vi "Mining Routine.vi"(9 "Blocks to find":i32=1, 10 "camera params":T4, 11 "FPGA VI Reference In":T1) -> (2 "Timed out":bool)   [LabVIEW 2012]
uses:
  <vilib>/vision/Image Controls.llb/IMAQ Image.ctl
  <vilib>/httpClient/ClientHandle.ctl
  FPGA_ref.ctl
  Globals.vi
  <vilib>/httpClient/LabVIEWHTTPClient.lvlib
panel:
  in  "Timeout (ms)":u32=120000
  in  "Block forward \ntime (10ms)":i32=300
  in  "Forward safe distance":dbl=0.35
  in  "No block distance":dbl=0.5
  in  "Block pickup distance":dbl=0.35
  in  "Block Y-Offset":dbl=400.0
  in  "Block X-Offset":dbl=160.0
  in  "Camera turn speed":dbl=0.25
  in  "Block Mid Range":dbl=50.0
  in  "no block turn speed":dbl=0.3
  # "Complete mining routine to search for & collect blocks\n\nWill exit when all blocks are found, or timeout occours"
  # "Not calibrated. Guessed.."
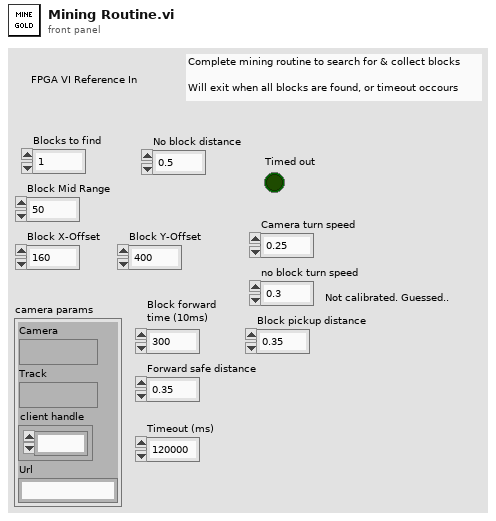
[diagram p1: front panel]
types:
  T1 = typedef "FPGA_ref.ctl" = refnum<k20>
  T2 = typedef "IMAQ Image.ctl" = refnum<image>
  T3 = typedef "LabVIEWHTTPClient.lvlib/ClientHandle.ctl" = refnum<k1>
  T4 = cluster{"Camera":T2, "Track":T2, "client handle":T3, "Url":string}
  T5 = cluster{"X Velocity (m/s)":dbl, "Y Velocity (m/s)":dbl, "Angular Velocity (rad/s)":dbl}
  T6 = cluster{"Blocks picked up":i32, "Timeout":i32, "Next state":enum16{"start", "find block", "align block", "pickup block", "sort block", "finish"}, "Future state":enum16{"start", "find block", "align block", "pickup block", "sort block", "finish"}, "Blocks to find":i32}
  T7 = enum16{"start", "find block", "align block", "pickup block", "sort block", "finish"}
  T8 = enum16{"position", "arm down", "forward", "grab", "arm up"}
  T9 = enum16{"wait", "open", "close", "lift", "lower", "pickup", "Flip", "UnFlip", "Latch", "UnLatch", "Setup"}
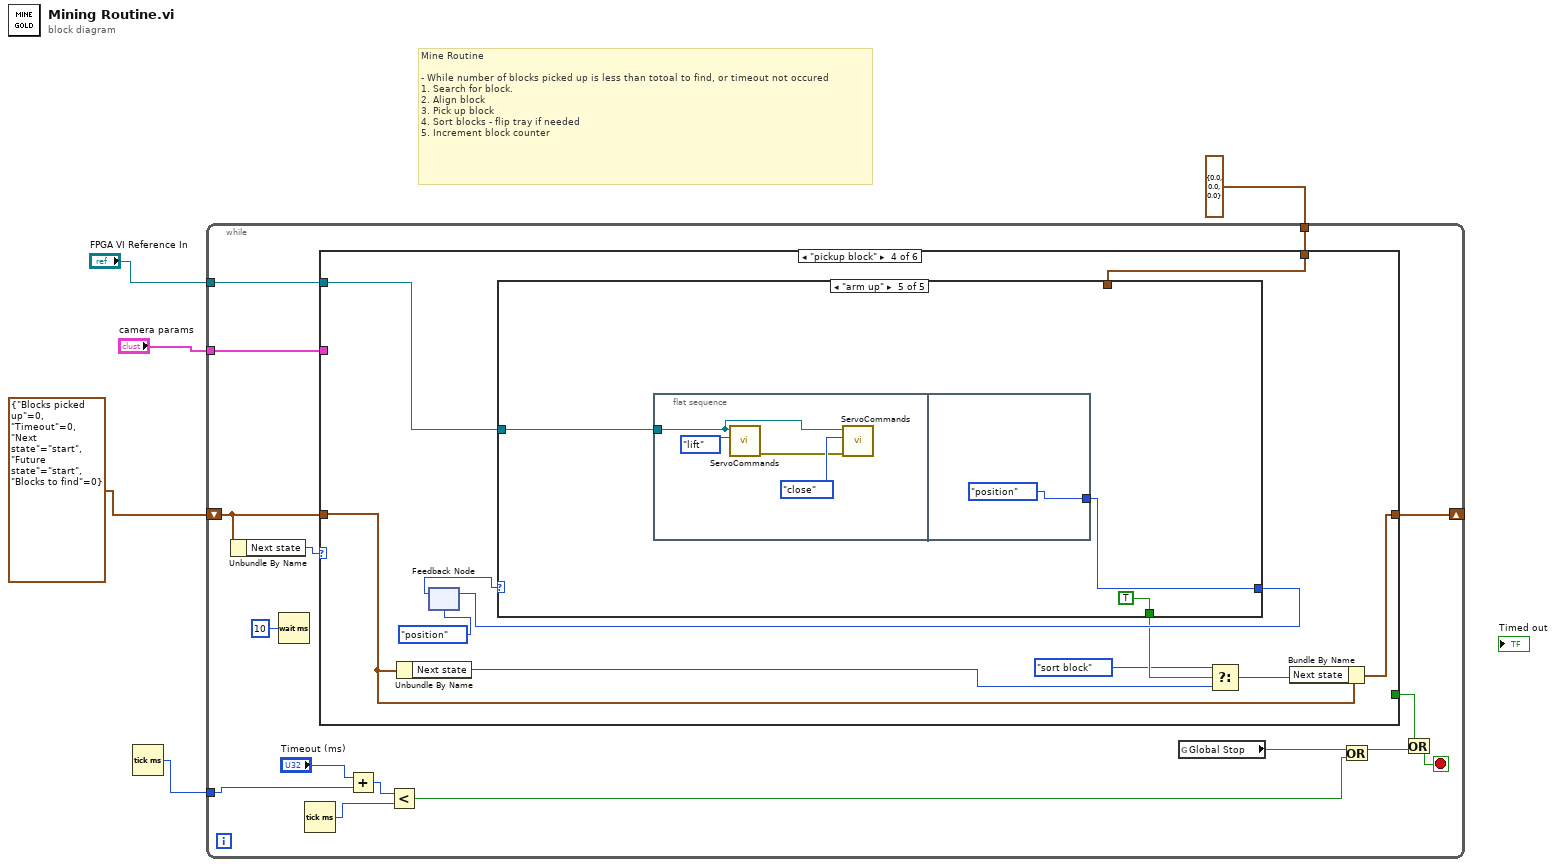
[diagram p0: block diagram]
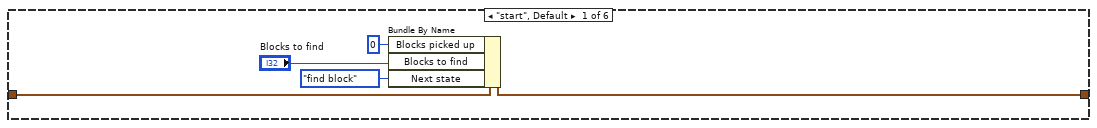
[diagram p2: hidden frame]
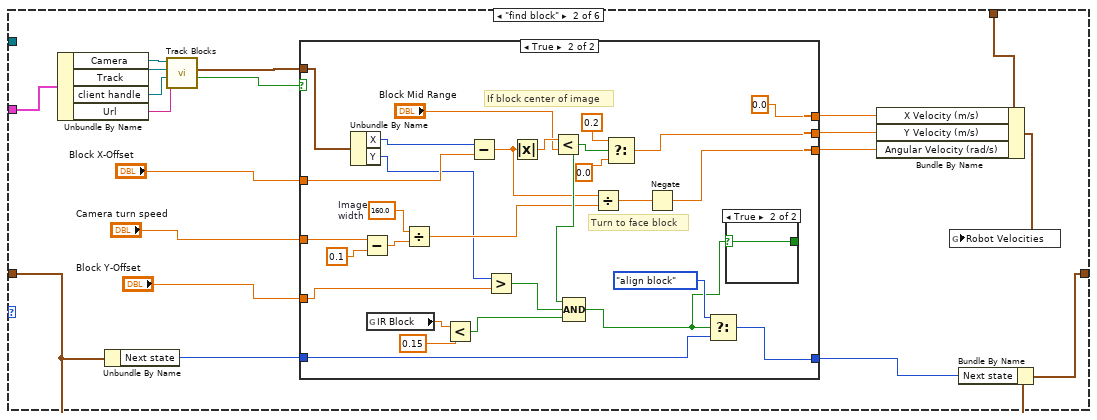
[diagram p3: hidden frame]
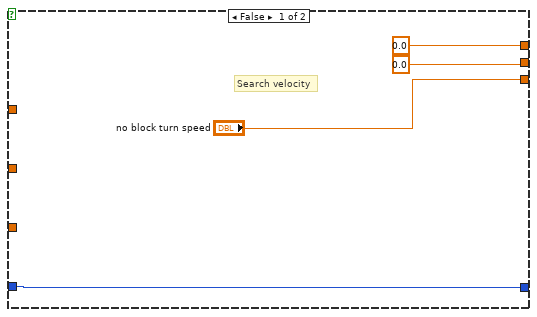
[diagram p4: hidden frame]
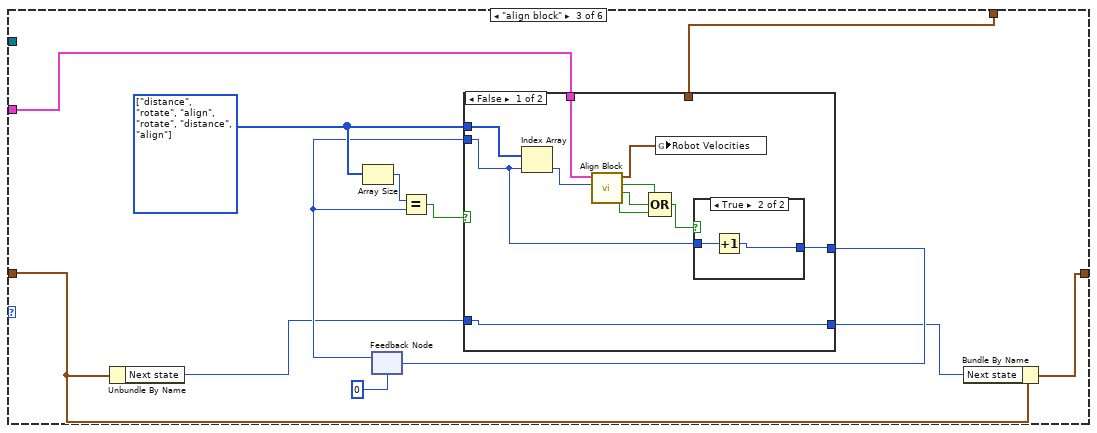
[diagram p6: hidden frame]
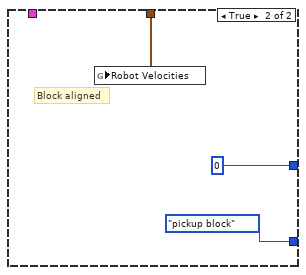
[diagram p8: hidden frame]
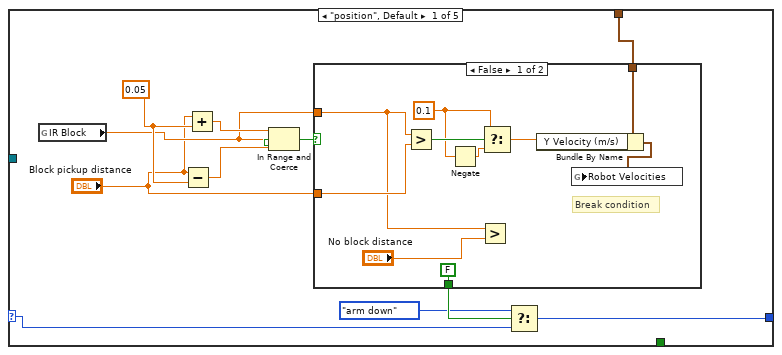
[diagram p9: hidden frame]
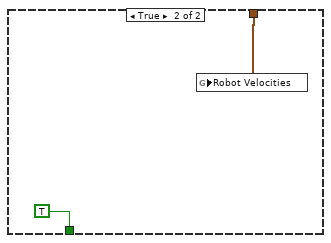
[diagram p10: hidden frame]
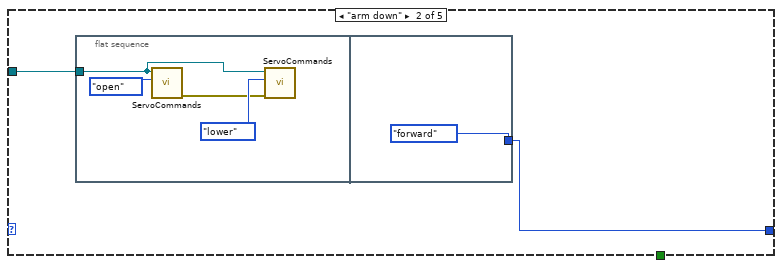
[diagram p11: hidden frame]
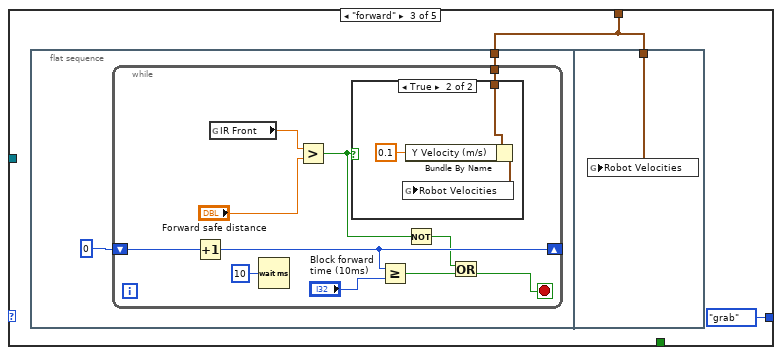
[diagram p12: hidden frame]
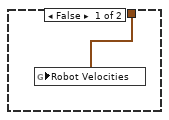
[diagram p13: hidden frame]
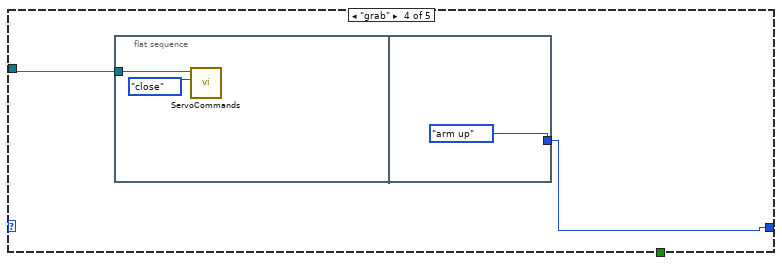
[diagram p14: hidden frame]
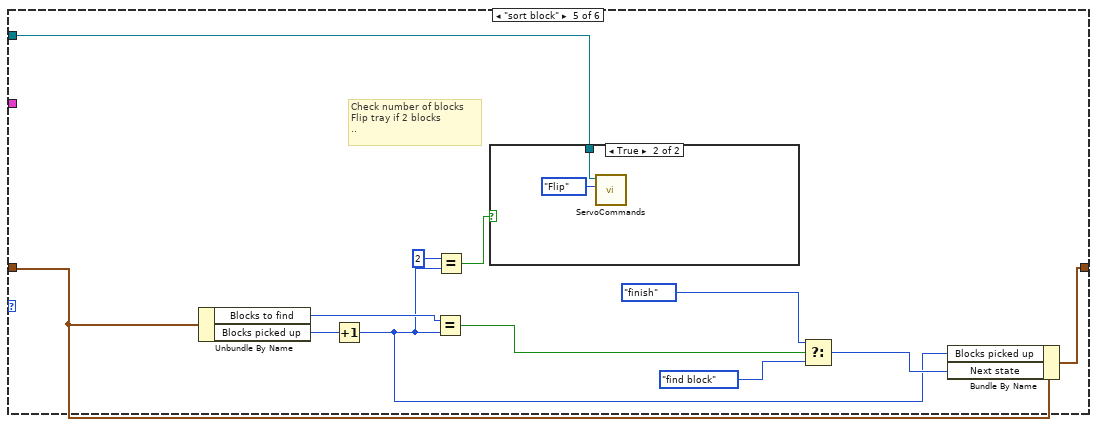
[diagram p15: hidden frame]
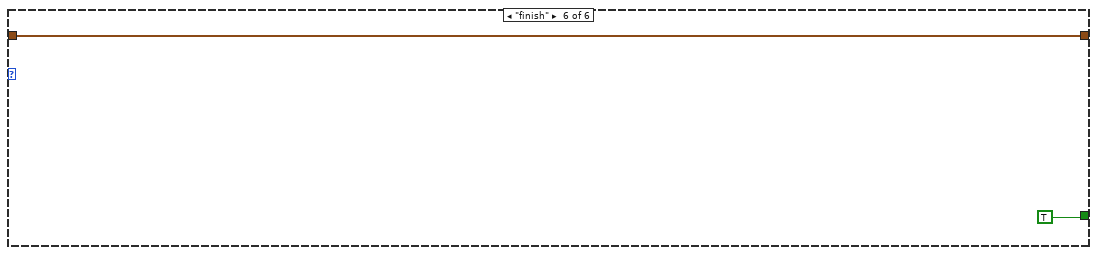
[diagram p17: hidden frame]
diagram:
  # "Mine Routine\n\n- While number of blocks picked up is less than totoal to find, or timeout not occured\n1. Search for block.\n2. Align block\n3. Pick up block\n4. Sort blocks - flip tray if needed\n5. Increment block counter"
  n1 = Tick Count (ms)() -> (millisecond timer value=w1:u32)
  n2 = while {
    shift-right: [w21] -> _
    shift-left: T6 {"Blocks picked up"=0, "Timeout"=0, "Next state"=enum."start", "Future state"=enum."start", "Blocks to find"=0} -> [w18]
    tunnel: T5 {"X Velocity (m/s)"=0.0, "Y Velocity (m/s)"=0.0, "Angular Velocity (rad/s)"=0.0} ("Robot Velocities") -> [w20]
    tunnel: "camera params" -> [w19]
    tunnel: "FPGA VI Reference In" -> [w15]
    tunnel: w1 -> [w11]
    stop <- w13 stop-if-true
    n3 = Unbundle By Name(w18) -> ("Next state"=w17:T7)
    n4 = Wait (ms)(milliseconds to wait=u32 10) -> ()  [unwired: 1 out]
    n5 = Tick Count (ms)() -> (millisecond timer value=w8:u32)
    n6 = case shown="\"pickup block\"" w17 {
      tunnel: w18 -> [w26 w28 w83 w119 w191 w197]
      tunnel: [w25 w29 w84 w118 w194 w197] -> w21
      tunnel: w20 -> [_ w34 w80 w117 _ _]
      tunnel: w19 -> [_ w32 w85 _ _ _]
      tunnel: [_ _ _ _ _ TRUE] -> w16
      tunnel: w15 -> [_ _ _ w114 w183 _]
      frame "start", Default {
        n7 = Bundle By Name(cluster=w26, "Blocks picked up"=0, "Blocks to find"="Blocks to find", "Next state"=T7."find block") -> (w25:T6)
      }
      frame "find block" {
        n8 = Unbundle By Name(w32) -> ("Camera"=w45:T2, "Track"=w44:T2, "client handle"=w38:T3, "Url"=w37:string)
        n9 = Unbundle By Name(w28) -> ("Next state"=w27:T7)
        n10 = call "Track Blocks.vi"("Url"=w37, "client handle"=w38, "Image Dst"=w44, "New Image"=w45) -> ("Object found?"=w39:bool, "Object Output"=w40:cluster{"X":i32, "Y":i32})  [unwired: 5 in, 1 out]
        n11 = case shown="True" w39 {
          tunnel: [0.0 ("X Velocity (m/s)") 0.0 ("X Velocity (m/s)")] -> w43
          tunnel: ["no block turn speed" w60] -> w42
          tunnel: [0.0 ("f") w76] -> w41
          tunnel: w40 -> [_ w73]
          tunnel: "Camera turn speed" -> [_ w65]
          tunnel: "Block X-Offset" -> [_ w66]
          tunnel: "Block Y-Offset" -> [_ w58]
          tunnel: [w46 w55] -> w30
          tunnel: w27 -> [w46 w54]
          frame False {
            # "Search velocity"
          }
          frame True {
            w62 = 160.0  # Image  width
            # "Turn to face block"
            # "If block center of image"
            n12 = Unbundle By Name(w73) -> ("X"=w68:i32, "Y"=w59:i32)
            n13 = Subtract(x=w65, y=0.1) -> (x-y=w63:dbl)
            n14 = global read "Globals.vi" "IR Block"() -> (w53:dbl)
            n15 = Divide(x=w62, y=w63) -> (x/y=w61:dbl)
            n16 = Less?(x=w53, y=0.15) -> (x < y?=w51:bool)
            n17 = Subtract(x=w68, y=w66) -> (x-y=w67:dbl)
            n18 = Greater?(x=w59, y=w58) -> (0:w57:bool)
            n19 = Absolute Value(x=w67) -> (abs(x)=w71:dbl)
            n20 = Less?(x=w71, y="Block Mid Range") -> (x < y?=w72:bool)
            n21 = Compound Arithmetic op=AND(w72, w57, w51) -> (w50:bool)
            n22 = Divide(x=w67, y=w61) -> (x/y=w69:dbl)
            n23 = Select(t=0.2, s=w72, f=0.0) -> (s? t:f=w76:dbl)
            n24 = Negate(x=w69) -> (-x=w60:dbl)
            n25 = Select(t=T7."align block" ("Next state"), s=w50, f=w54) -> (s? t:f=w55:T7)
            n26 = case shown="True" w50 {
              selector: w50 -> [w78 w79]
              tunnel: [w78 w79] -> _
              frame False {
              }
              frame True {
              }
            }
          }
        }
        n27 = Bundle By Name(cluster=w34, "X Velocity (m/s)"=w43, "Y Velocity (m/s)"=w41, "Angular Velocity (rad/s)"=w42) -> (w33:T5)
        n28 = global write "Globals.vi" "Robot Velocities"(w33) -> ()
        n29 = Bundle By Name(cluster=w28, "Next state"=w30) -> (w29:T6)
      }
      frame "align block" {
        w91 = enum16{"distance", "align", "rotate"}[] [enum."distance", enum."rotate", enum."align", enum."rotate", enum."distance", enum."align"] items=["distance", "align", "rotate"]
        n30 = Unbundle By Name(w83) -> ("Next state"=w82:T7)
        n31 = Array Size(array=w91) -> (size(s)=w89:i32)
        n32 = feedback #1(0) -> (w86:i32)
        n33 = Equal?(x=w89, y=w86) -> (x = y?=w88:bool)
        n34 = case shown="False" w88 {
          tunnel: w85 -> [w101 _]
          tunnel: w91 -> [w100 _]
          tunnel: w86 -> [w96 _]
          tunnel: [w95 0] -> w87
          tunnel: w82 -> [w92 _]
          tunnel: [w92 T7."pickup block"] -> w81
          tunnel: w80 -> [_ w106]
          frame False {
            n35 = Index Array(array=w100, index=w96) -> (element=w102:enum16{"distance", "align", "rotate"})
            n36 = call "Align Block.vi"("Command"=w102, "Camera In"=w101) -> ("Block orientated?"=w93:bool, "Block centered?"=w97:bool, "Block in front?"=w98:bool, "Robot Velocities"=w94:T5)  [unwired: 6 in]
            n37 = Compound Arithmetic op=OR(w98, w97, w93) -> (w99:bool)
            n38 = global write "Globals.vi" "Robot Velocities"(w94) -> ()
            n39 = case shown="True" w99 {
              tunnel: w96 -> [w103 w105]
              tunnel: [w103 w104] -> w95
              frame False {
              }
              frame True {
                n40 = Increment(x=w105) -> (x+1=w104:i32)
              }
            }
          }
          frame True {
            # "Block aligned"
            n41 = global write "Globals.vi" "Robot Velocities"(w106) -> ()
          }
        }
        n42 = feedback-in #1(w87) -> ()
        n43 = Bundle By Name(cluster=w83, "Next state"=w81) -> (w84:T6)
      }
      frame "pickup block" {
        n44 = Unbundle By Name(w119) -> ("Next state"=w115:T7)
        n45 = feedback #2(T8."position") -> (w112:T8)
        n46 = case shown="\"arm up\"" w112 {
          selector: w112 -> [w123 _ _ _ _]
          tunnel: w117 -> [w124 _ w150 _ _]
          tunnel: w114 -> [_ w144 _ w171 w177]
          tunnel: [w121 w143 T8."grab" w170 w176] -> w111
          tunnel: [_ _ _ _ TRUE] -> w110
          frame "position", Default {
            w127 = 0.05
            n47 = global read "Globals.vi" "IR Block"() -> (w126:dbl)
            n48 = Subtract(x="Block pickup distance", y=w127) -> (x-y=w128:dbl)
            n49 = Add(x="Block pickup distance", y=w127) -> (x+y=w129:dbl)
            n50 = In Range and Coerce(upper limit=w129, x=w126, lower limit=w128) -> (In Range?=w130:bool)  [unwired: 1 out]
            n51 = case shown="False" w130 {
              tunnel: w126 -> [w135 _]
              tunnel: "Block pickup distance" -> [w140 _]
              tunnel: w124 -> [w133 w142]
              tunnel: [FALSE TRUE] -> w122
              frame False {
                w136 = 0.1 ("t")
                # "Break condition"
                n52 = Greater?(x=w135, y=w140) -> (0:w139:bool)
                n53 = Negate(x=w136) -> (-x=w137:dbl)
                n54 = Greater?(x=w135, y="No block distance") -> ()  [unwired: 1 out]
                n55 = Select(t=w136, s=w139, f=w137) -> (s? t:f=w138:dbl)
                n56 = Bundle By Name(cluster=w133, "Y Velocity (m/s)"=w138) -> (w132:T5)
                n57 = global write "Globals.vi" "Robot Velocities"(w132) -> ()
              }
              frame True {
                n58 = global write "Globals.vi" "Robot Velocities"(w142) -> ()
              }
            }
            n59 = Select(t=T8."arm down", s=w122, f=w123) -> (s? t:f=w121:T8)
          }
          frame "arm down" {
            n60 = flat-sequence {
              tunnel: w144 -> [w145]
              tunnel: [T8."forward"] -> w143
              frame #0 {
                n61 = call "ServoCommands.vi"("State"=T9."open", "FPGA VI Reference In"=w145) -> ("error out"=w146:errorcluster)  [unwired: 9 in]
                n62 = call "ServoCommands.vi"("error in"=w146, "State"=T9."lower", "FPGA VI Reference In"=w145) -> ()  [unwired: 8 in, 1 out]
              }
              frame #1 {
              }
            }
          }
          frame "forward" {
            n63 = flat-sequence {
              tunnel: w150 -> [w153]
              tunnel: w150 -> [w169]
              frame #0 {
                n64 = while {
                  tunnel: w153 -> [w162]
                  shift-right: [w160] -> _
                  shift-left: 0 -> [w161]
                  stop <- w157 stop-if-true
                  n65 = Increment(x=w161) -> (x+1=w160:i32)
                  n66 = global read "Globals.vi" "IR Front"() -> (w164:dbl)
                  n67 = Wait (ms)(milliseconds to wait=u32 10) -> ()  [unwired: 1 out]
                  n68 = Greater?(x=w164, y="Forward safe distance") -> (0:w156:bool)
                  n69 = case shown="True" w156 {
                    tunnel: w162 -> [w165 w168]
                    frame False {
                      n70 = global write "Globals.vi" "Robot Velocities"(w165) -> ()
                    }
                    frame True {
                      n71 = Bundle By Name(cluster=w168, "Y Velocity (m/s)"=0.1) -> (w167:T5)
                      n72 = global write "Globals.vi" "Robot Velocities"(w167) -> ()
                    }
                  }
                  n73 = Greater Or Equal?(x=w160, y="Block forward \ntime (10ms)") -> (x >= y?=w158:bool)
                  n74 = Not(x=w156) -> (.not. x?=w155:bool)
                  n75 = Or(x=w155, y=w158) -> (x .or. y?=w157:bool)
                }
              }
              frame #1 {
                n76 = global write "Globals.vi" "Robot Velocities"(w169) -> ()
              }
            }
          }
          frame "grab" {
            n77 = flat-sequence {
              tunnel: w171 -> [w172]
              tunnel: [T8."arm up"] -> w170
              frame #0 {
                n78 = call "ServoCommands.vi"("State"=T9."close", "FPGA VI Reference In"=w172) -> ()  [unwired: 9 in, 1 out]
              }
              frame #1 {
              }
            }
          }
          frame "arm up" {
            n79 = flat-sequence {
              tunnel: w177 -> [w178]
              tunnel: [T8."position"] -> w176
              frame #0 {
                n80 = call "ServoCommands.vi"("State"=T9."lift", "FPGA VI Reference In"=w178) -> ("error out"=w179:errorcluster)  [unwired: 9 in]
                n81 = call "ServoCommands.vi"("error in"=w179, "State"=T9."close", "FPGA VI Reference In"=w178) -> ()  [unwired: 8 in, 1 out]
              }
              frame #1 {
              }
            }
          }
        }
        n82 = feedback-in #2(w111) -> ()
        n83 = Select(t=T7."sort block", s=w110, f=w115) -> (s? t:f=w116:T7)
        n84 = Bundle By Name(cluster=w119, "Next state"=w116) -> (w118:T6)
      }
      frame "sort block" {
        # "Check number of blocks\nFlip tray if 2 blocks\n.."
        n85 = Unbundle By Name(w191) -> ("Blocks to find"=w190:i32, "Blocks picked up"=w187:i32)
        n86 = Increment(x=w187) -> (x+1=w186:i32)
        n87 = Equal?(x=w190, y=w186) -> (x = y?=w189:bool)
        n88 = Equal?(x=2, y=w186) -> (x = y?=w184:bool)
        n89 = case shown="True" w184 {
          tunnel: w183 -> [_ w196]
          frame False {
          }
          frame True {
            n90 = call "ServoCommands.vi"("State"=T9."Flip", "FPGA VI Reference In"=w196) -> ()  [unwired: 9 in, 1 out]
          }
        }
        n91 = Select(t=T7."finish" ("Next state"), s=w189, f=T7."find block") -> (s? t:f=w193:T7)
        n92 = Bundle By Name(cluster=w191, "Blocks picked up"=w186, "Next state"=w193) -> (w194:T6)
      }
      frame "finish" {
      }
    }
    n93 = Add(x="Timeout (ms)", y=w11) -> (x+y=w10:u32)
    n94 = Less?(x=w10, y=w8) -> (x < y?=w6:bool)
    n95 = global read "Globals.vi" "Global Stop"() -> (w12:bool)
    n96 = Or(x=w12, y=w6) -> (x .or. y?=w7:bool)
    n97 = Or(x=w16, y=w7) -> (x .or. y?=w13:bool)
  }
